vi "Arc Mode Select.vi"(1 "Angle":dbl) -> (0 "Mode":u8)   [LabVIEW 2012, in "ProcessorHelperFunctions.lvlib"]
uses:
  ProcessorHelperFunctions.lvlib
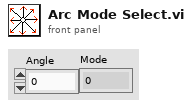
[diagram p1: front panel]
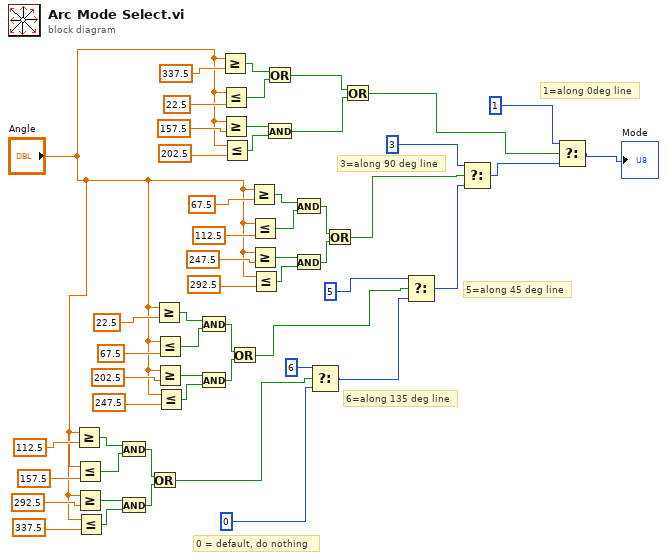
[diagram p0: block diagram]
diagram:
  # "0 = default, do nothing"
  # "6=along 135 deg line"
  # "5=along 45 deg line"
  # "3=along 90 deg line"
  # "1=along 0deg line"
  n1 = Greater Or Equal?(x="Angle", y=112.5) -> (x >= y?=w11:bool)
  n2 = Less Or Equal?(x="Angle", y=157.5) -> (x <= y?=w10:bool)
  n3 = Greater Or Equal?(x="Angle", y=292.5) -> (x >= y?=w6:bool)
  n4 = Less Or Equal?(x="Angle", y=337.5) -> (x <= y?=w5:bool)
  n5 = And(x=w11, y=w10) -> (x .and. y?=w4:bool)
  n6 = And(x=w6, y=w5) -> (x .and. y?=w3:bool)
  n7 = Or(x=w4, y=w3) -> (x .or. y?=w1:bool)
  n8 = Greater Or Equal?(x="Angle", y=22.5) -> (x >= y?=w22:bool)
  n9 = Less Or Equal?(x="Angle", y=67.5) -> (x <= y?=w21:bool)
  n10 = Greater Or Equal?(x="Angle", y=202.5) -> (x >= y?=w17:bool)
  n11 = Less Or Equal?(x="Angle", y=247.5) -> (x <= y?=w16:bool)
  n12 = And(x=w22, y=w21) -> (x .and. y?=w15:bool)
  n13 = And(x=w17, y=w16) -> (x .and. y?=w14:bool)
  n14 = Greater Or Equal?(x="Angle", y=337.5) -> (x >= y?=w52:bool)
  n15 = Less Or Equal?(x="Angle", y=22.5) -> (x <= y?=w51:bool)
  n16 = Greater Or Equal?(x="Angle", y=157.5) -> (x >= y?=w44:bool)
  n17 = Less Or Equal?(x="Angle", y=202.5) -> (x <= y?=w43:bool)
  n18 = Or(x=w15, y=w14) -> (x .or. y?=w13:bool)
  n19 = Greater Or Equal?(x="Angle", y=67.5) -> (x >= y?=w38:bool)
  n20 = Less Or Equal?(x="Angle", y=112.5) -> (x <= y?=w37:bool)
  n21 = Greater Or Equal?(x="Angle", y=247.5) -> (x >= y?=w33:bool)
  n22 = Less Or Equal?(x="Angle", y=292.5) -> (x <= y?=w32:bool)
  n23 = Or(x=w52, y=w51) -> (x .or. y?=w41:bool)
  n24 = And(x=w44, y=w43) -> (x .and. y?=w42:bool)
  n25 = And(x=w38, y=w37) -> (x .and. y?=w31:bool)
  n26 = And(x=w33, y=w32) -> (x .and. y?=w30:bool)
  n27 = Select(t=6, s=w1, f=0) -> (s? t:f=w25:i32)
  n28 = Or(x=w31, y=w30) -> (x .or. y?=w29:bool)
  n29 = Or(x=w41, y=w42) -> (x .or. y?=w40:bool)
  n30 = Select(t=5, s=w13, f=w25) -> (s? t:f=w28:i32)
  n31 = Select(t=3, s=w29, f=w28) -> (s? t:f=w48:i32)
  n32 = Select(t=1, s=w40, f=w48) -> (s? t:f=→"Mode":i32)
